vi "Mechanical Shutter Module.vi"(7 "Actions":T1=enum."Clear", 8 "Error In":errorcluster, 11 "Mech. Shutter Status [In]":enum16{"Close", "Open"}(ring)) -> (0 "Error Out":errorcluster, 3 "Mech. Shutter Status [Out]":enum16{"Close", "Open"}(ring))   [LabVIEW 2018]
uses:
  General/Controls/FGV Actions.ctl
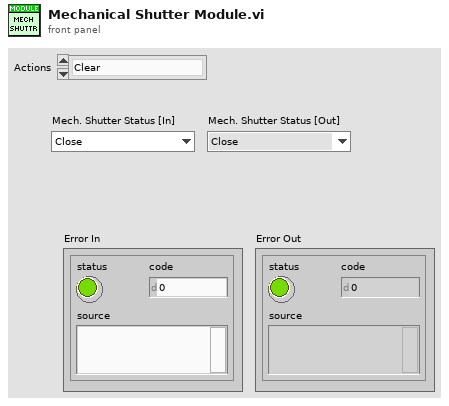
[diagram p1: front panel]
types:
  T1 = typedef "FGV Actions.ctl" = enum16{"Init", "Set", "Get", "Clear"}
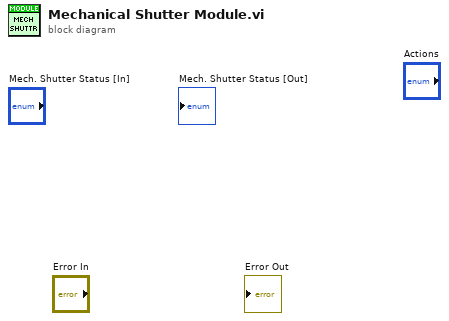
[diagram p0: block diagram]
diagram:
